vi "Merge BMP.vi"(1 "image two":T1, 2 "image one":T1) -> (0 "Merged":T1)   [LabVIEW 2022 SP3]
uses:
  <vilib>/picture/picture.llb/imagedata.ctl
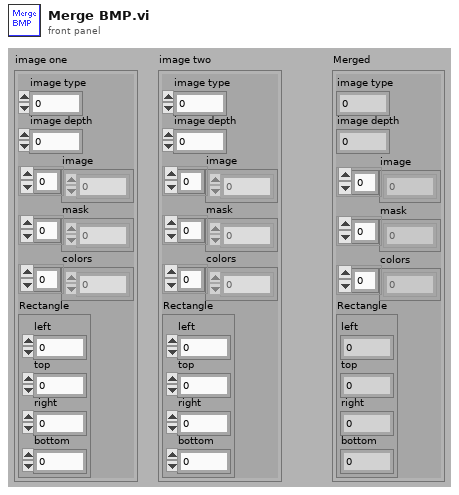
[diagram p1: front panel]
types:
  T1 = typedef "imagedata.ctl" = cluster{"image type":i32, "image depth":i32, "image":u8[], "mask":u8[], "colors":u32[], "Rectangle":cluster{"left":i16, "top":i16, "right":i16, "bottom":i16}}
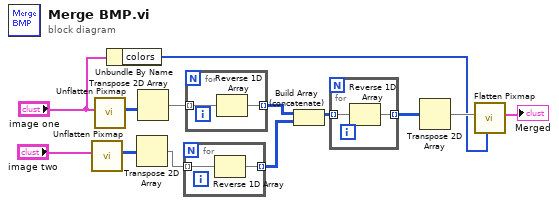
[diagram p0: block diagram]
diagram:
  n1 = call <vilib>:"Unflatten Pixmap.vi"("image data"="image two") -> ("8-bit pixmap"=w7:u8[][])  [unwired: 10 out]
  n2 = call <vilib>:"Unflatten Pixmap.vi"("image data"="image one") -> ("8-bit pixmap"=w6:u8[][])  [unwired: 10 out]
  n3 = Unbundle By Name("image one") -> ("colors"=w4:u32[])
  n4 = Transpose 2D Array(2D array=w7) -> (transposed array=w12:u8[][])
  n5 = Transpose 2D Array(2D array=w6) -> (transposed array=w5:u8[][])
  n6 = for {
    tunnel: w12 -> [w15] mode=indexing
    tunnel: [w14] -> w13 mode=indexing
    n7 = Reverse 1D Array(array=w15) -> (reversed array=w14:u8[])
  }
  n8 = for {
    tunnel: w5 -> [w17] mode=indexing
    tunnel: [w16] -> w10 mode=indexing
    n9 = Reverse 1D Array(array=w17) -> (reversed array=w16:u8[])
  }
  n10 = Build Array (concatenate)(w10, w13) -> (w8:u8[][])
  n11 = for {
    tunnel: [w19] -> w9 mode=indexing
    tunnel: w8 -> [w18] mode=indexing
    n12 = Reverse 1D Array(array=w18) -> (reversed array=w19:u8[])
  }
  n13 = Transpose 2D Array(2D array=w9) -> (transposed array=w11:u8[][])
  n14 = call <vilib>:"Flatten Pixmap.vi"("colors"=w4, "8-bit pixmap"=w11) -> ("image data"=→"Merged":T1)  [unwired: 4 in, 5 out]
